vi "ep_Order Waveform and Set Attributes.vi"(0 "voltage channels":T1[](array[typedef]) {"physical channels"."channel phase" items=["Phase A (L1)", "Phase B (L2)", "Phase C (L3)", "Phase N (Neutral)"]}, 5 "current channels":T1[](array[typedef]) {"physical channels"."channel phase" items=["Phase A (L1)", "Phase B (L2)", "Phase C (L3)", "Phase N (Neutral)"]}, 7 "reset? (F)":bool, 11 "error in (no error)":errorcluster) -> (4 "voltage waveforms":waveform(sgl)[](array[waveform]), 6 "voltage physical channel indexes":u16[](array[numeric]), 8 "current waveforms":waveform(sgl)[](array[waveform]), 10 "current physical channel indexes":u16[](array[numeric]), 15 "error out":errorcluster)   [LabVIEW 2014, in "NI_EP_Power Quality.lvlib"]
uses:
  <vilib>/addons/Electrical Power/PQ/NI_EP_Power Quality.lvlib
  <vilib>/addons/Electrical Power/PQ/Common/Controls/ep_Channels Config.ctl
  <vilib>/addons/Electrical Power/PQ/Common/Controls/ep_Channel Phase.ctl
  <vilib>/addons/Electrical Power/PQ/Common/Controls/ep_AI Data Channel.ctl
panel:
  in  "waveform":waveform(sgl)
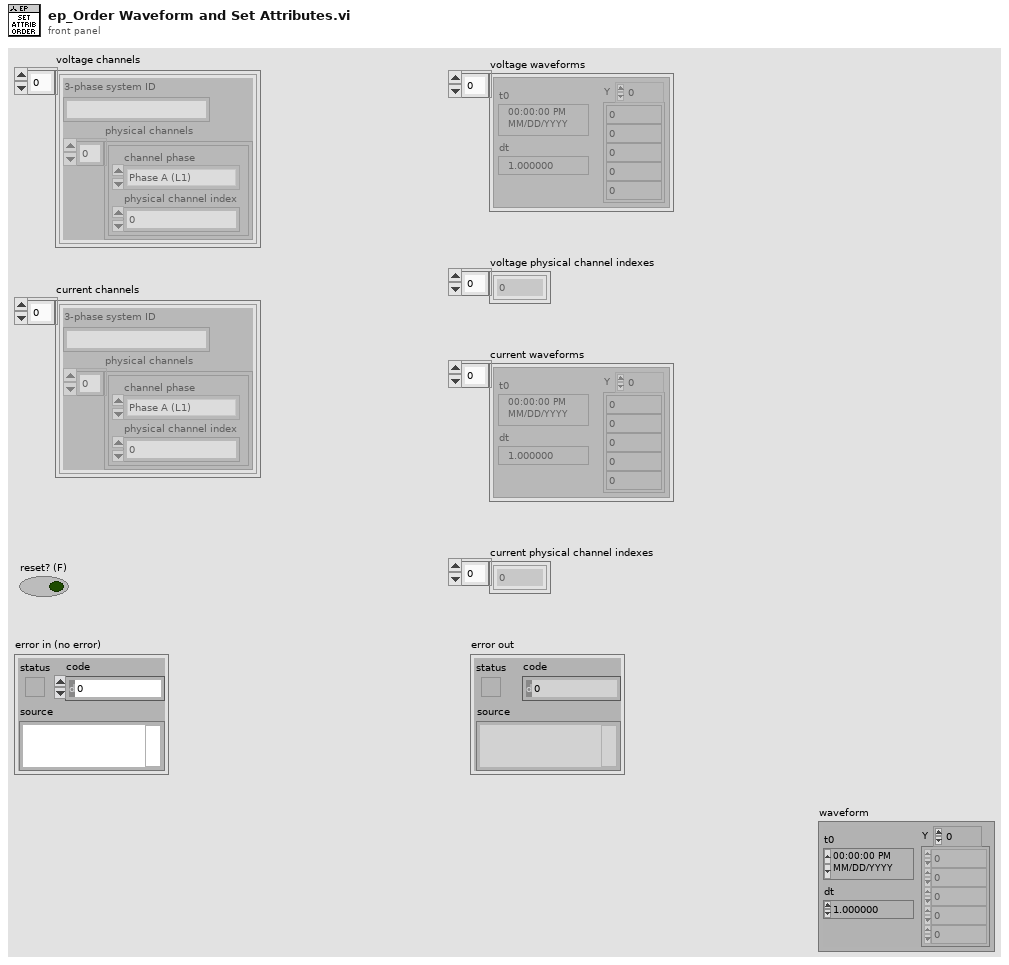
[diagram p1: front panel]
types:
  T1 = typedef "NI_EP_Power Quality.lvlib/ep_Channels Config.ctl" = cluster{"3-phase system ID":string, "physical channels":cluster{"channel phase":T2, "physical channel index":u16}[]}
  T2 = typedef "NI_EP_Power Quality.lvlib/ep_Channel Phase.ctl" = u16
  T3 = typedef "NI_EP_Power Quality.lvlib/ep_AI Data Channel.ctl" = enum16{"Voltage Phase A (L1)", "Voltage Phase B (L2)", "Voltage Phase C (L3)", "Voltage Phase N (Neutral)", "Current Phase A (L1)", "Current Phase B (L2)", "Current Phase C (L3)", "Current Phase N (Neutral)"}
  T4 = cluster{"channel phase":T2, "physical channel index":u16}[]
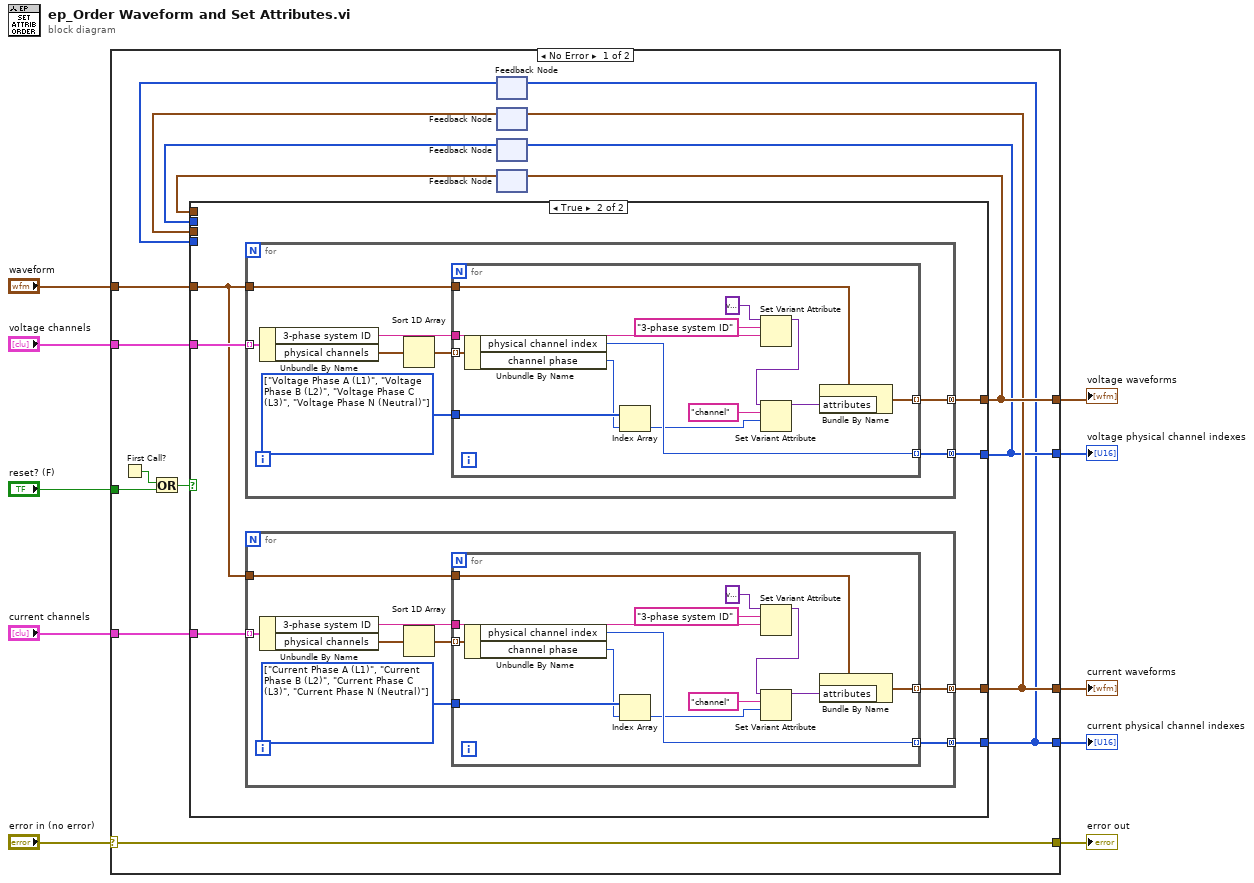
[diagram p0: block diagram]
diagram:
  n1 = case shown="No Error" "error in (no error)" {
    selector: "error in (no error)" -> [w14 w79]
    tunnel: "voltage channels" -> [w25 _]
    tunnel: "waveform" -> [w24 _]
    tunnel: "current channels" -> [w23 _]
    tunnel: [w22 _] -> w9
    tunnel: [w21 _] -> w8
    tunnel: [w18 _] -> w7
    tunnel: [w16 _] -> w6
    tunnel: "reset? (F)" -> [w12 _]
    tunnel: [w14 w79] -> w3
    frame No Error {
      n2 = First Call?() -> (First Call?: T/F=w11:bool)
      n3 = Or(x=w11, y=w12) -> (x .or. y?=w13:bool)
      n4 = feedback #1() -> (w15:u16[])  [unwired: 1 in]
      n5 = feedback #2() -> (w19:waveform(sgl)[])  [unwired: 1 in]
      n6 = feedback #3() -> (w17:u16[])  [unwired: 1 in]
      n7 = feedback #4() -> (w20:waveform(sgl)[])  [unwired: 1 in]
      n8 = case shown="True" w13 {
        tunnel: w25 -> [_ w36]
        tunnel: w24 -> [_ w33]
        tunnel: w23 -> [_ w32]
        tunnel: [w29 w35] -> w22
        tunnel: [w28 w31] -> w21
        tunnel: w20 -> [w29 _]
        tunnel: w19 -> [w28 _]
        tunnel: [w27 w34] -> w18
        tunnel: [w26 w30] -> w16
        tunnel: w17 -> [w27 _]
        tunnel: w15 -> [w26 _]
        frame False {
        }
        frame True {
          n9 = for {
            tunnel: w36 -> [w65] mode=indexing
            tunnel: w33 -> [w62]
            tunnel: [w60] -> w35 mode=concatenating
            tunnel: [w59] -> w34 mode=concatenating
            w58 = T3[] [enum."Voltage Phase A (L1)", enum."Voltage Phase B (L2)", enum."Voltage Phase C (L3)", enum."Voltage Phase N (Neutral)"] items=["Voltage Phase A (L1)", "Voltage Phase B (L2)", "Voltage Phase C (L3)", "Voltage Phase N (Neutral)", "Current Phase A (L1)", "Current Phase B (L2)", "Current Phase C (L3)", "Current Phase N (Neutral)"]
            n10 = Unbundle By Name(w65) -> ("3-phase system ID"=w61:string, "physical channels"=w64:T4)
            n11 = Sort 1D Array(array=w64) -> (sorted array=w63:T4)
            n12 = for {
              tunnel: w63 -> [w77] mode=indexing
              tunnel: w62 -> [w70]
              tunnel: w61 -> [w74]
              tunnel: [w71] -> w60 mode=indexing
              tunnel: [w73] -> w59 mode=indexing
              tunnel: w58 -> [w69]
              n13 = Unbundle By Name(w77) -> ("physical channel index"=w73:u16, "channel phase"=w68:T2)
              n14 = Index Array(array=w69, index=w68) -> (element=w67:T3)
              n15 = Set Variant Attribute(Variant=variant ("variant"), name="3-phase system ID", value=w74) -> (Variant out=w66:variant)  [unwired: 1 in, 2 out]
              n16 = Set Variant Attribute(Variant=w66, name="channel", value=w67) -> (Variant out=w72:variant)  [unwired: 1 in, 2 out]
              n17 = Bundle By Name(cluster=w70, "attributes"=w72) -> (w71:waveform(sgl))
            }
          }
          n18 = for {
            tunnel: w32 -> [w44] mode=indexing
            tunnel: w33 -> [w41]
            tunnel: [w39] -> w31 mode=concatenating
            tunnel: [w38] -> w30 mode=concatenating
            w37 = T3[] [enum."Current Phase A (L1)", enum."Current Phase B (L2)", enum."Current Phase C (L3)", enum."Current Phase N (Neutral)"] items=["Voltage Phase A (L1)", "Voltage Phase B (L2)", "Voltage Phase C (L3)", "Voltage Phase N (Neutral)", "Current Phase A (L1)", "Current Phase B (L2)", "Current Phase C (L3)", "Current Phase N (Neutral)"]
            n19 = Unbundle By Name(w44) -> ("3-phase system ID"=w40:string, "physical channels"=w43:T4)
            n20 = Sort 1D Array(array=w43) -> (sorted array=w42:T4)
            n21 = for {
              tunnel: w42 -> [w56] mode=indexing
              tunnel: w41 -> [w49]
              tunnel: w40 -> [w53]
              tunnel: [w50] -> w39 mode=indexing
              tunnel: [w52] -> w38 mode=indexing
              tunnel: w37 -> [w48]
              n22 = Unbundle By Name(w56) -> ("physical channel index"=w52:u16, "channel phase"=w47:T2)
              n23 = Index Array(array=w48, index=w47) -> (element=w46:T3)
              n24 = Set Variant Attribute(Variant=variant ("variant"), name="3-phase system ID", value=w53) -> (Variant out=w45:variant)  [unwired: 1 in, 2 out]
              n25 = Set Variant Attribute(Variant=w45, name="channel", value=w46) -> (Variant out=w51:variant)  [unwired: 1 in, 2 out]
              n26 = Bundle By Name(cluster=w49, "attributes"=w51) -> (w50:waveform(sgl))
            }
          }
        }
      }
      n27 = feedback-in #1(w16) -> ()
      n28 = feedback-in #2(w21) -> ()
      n29 = feedback-in #3(w18) -> ()
      n30 = feedback-in #4(w22) -> ()
    }
    frame Error {
    }
  }
  "error out" <- w3
  "voltage waveforms" <- w9
  "voltage physical channel indexes" <- w7
  "current waveforms" <- w8
  "current physical channel indexes" <- w6
